vi "AlliGator Plot Selected Global Fit Parameters.vi"(4 "R2 & RMSE":dbl[](array[numeric]), 6 "Global Fit Parameter Info":T1, 8 "error in (no error)":errorcluster, 9 "Best Fit Parameters":dbl[](array[numeric]), 10 "# Decays":i32, 11 "XYGraph in":refnum<vi>) -> (0 "error out":errorcluster)   [LabVIEW 2021, in "AlliGator Global Decay Fit.lvlib"]
uses:
  AlliGator Global Decay Fit.lvlib
  Fits/Global Fits/Global Fit Parameters Information.ctl
  Fits/Fits.lvlib
  Graphs/XY Graph/XY Graph Add-Ons.lvlib
  Decay Fit/AlliGator Decay Fit.lvlib
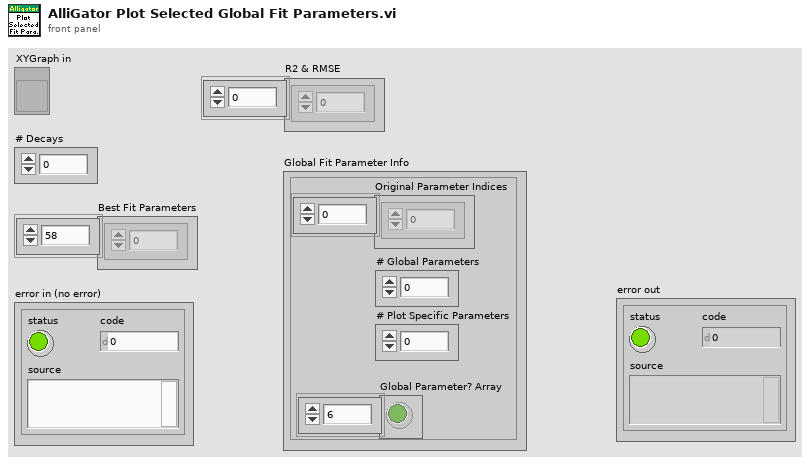
[diagram p1: front panel]
types:
  T1 = typedef "Fits.lvlib/Global Fit Parameters Information.ctl" = cluster{"Original Parameter Indices":i32[], "# Global Parameters":i32, "# Plot Specific Parameters":i32, "Global Parameter? Array":bool[]}
  T2 = typedef "AlliGator Decay Fit.lvlib/AlliGator Decay Fit Output Options.ctl" = cluster{"Fit Model":T3, "Decay Fit Parameter Array":T4[]}
  T3 = typedef "Fits.lvlib/Decay Model.ctl" = enum16{"1-Exponential", "2-Exponentials"}
  T4 = typedef "Fits.lvlib/Decay Fit Parameters & Derived Quantities List v2.ctl" = enum16{"Offset", "Baseline", "A_1", "tau_1", "A_2", "tau_2", "<tau>_a", "f1_a", "f2_a", "<tau>_i", "f1_i", "f2_i", "-", "R^2", "Chi^2"}
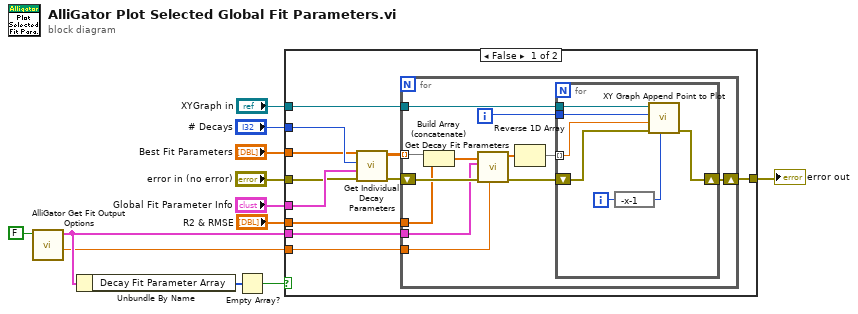
[diagram p0: block diagram]
diagram:
  n1 = call "AlliGator Get Fit Output Options.vi"("All Parameters?"=FALSE) -> ("Laser Period"=w1:dbl, "Decay Fit Output Options"=w2:T2)  [unwired: 8 in, 1 out]
  n2 = Unbundle By Name(w2) -> ("Decay Fit Parameter Array"=w4:T4[])
  n3 = Empty Array?(array=w4) -> (empty?=w3:bool)
  n4 = case shown="False" w3 {
    tunnel: "Global Fit Parameter Info" -> [w23 _]
    tunnel: "# Decays" -> [w22 _]
    tunnel: "Best Fit Parameters" -> [w21 _]
    tunnel: "error in (no error)" -> [w20 w42]
    tunnel: "XYGraph in" -> [w18 _]
    tunnel: [w16 w42] -> w7
    tunnel: "R2 & RMSE" -> [w15 _]
    tunnel: w2 -> [w14 _]
    tunnel: w1 -> [w13 _]
    frame False {
      n5 = call "Get Individual Decay Parameters.vi"("Error In"=w20, "Global Fit Parameter Info"=w23, "# Decays"=w22, "Global Fit Parameters Array"=w21) -> ("Error Out"=w17:errorcluster, "All Parameters Array"=w19:dbl[][])  [unwired: 4 in, 2 out]
      n6 = for {
        tunnel: w19 -> [w34] mode=indexing
        tunnel: w18 -> [w32]
        shift-right: [w29] -> w16
        shift-left: w17 -> [w30]
        tunnel: w15 -> [w27]
        tunnel: w14 -> [w25]
        tunnel: w13 -> [w24]
        i -> [w26]
        n7 = Build Array (concatenate)(w34, w27) -> (w28:dbl[])
        n8 = call "Get Decay Fit Parameters.vi"("Laser Period"=w24, "Decay Fit Output Options"=w25, "Decay Fit Parameters"=w28) -> ("Displayed Decay Fits Parameters"=w33:dbl[])  [unwired: 7 in, 1 out]
        n9 = Reverse 1D Array(array=w33) -> (reversed array=w31:dbl[])
        n10 = for {
          tunnel: w32 -> [w41]
          tunnel: w31 -> [w40] mode=indexing
          shift-right: [w37] -> w29
          shift-left: w30 -> [w38]
          tunnel: w26 -> [w35]
          i -> [w36]
          n11 = expression code="-x-1"(w36) -> (w39:i32)
          n12 = call "XY Graph Append Point to Plot.vi"("Plot ID (-1: last)"=w39, "error in (no error)"=w38, "y"=w40, "x"=w35, "XYGraph in"=w41) -> ("error out"=w37:errorcluster)  [unwired: 3 in, 3 out]
        }
      }
    }
    frame True {
    }
  }
  "error out" <- w7
